vi "_Hightlight CSM Scripts(StringConstant).vi"(11 "reference out":refnum<vi>) -> (0 "error out":errorcluster)   [LabVIEW 2017]
uses:
  Communicable State Machine.lvlib
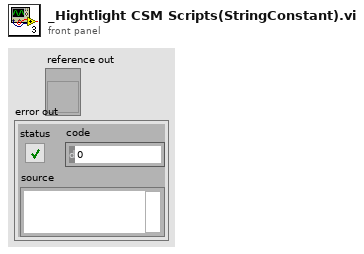
[diagram p1: front panel]
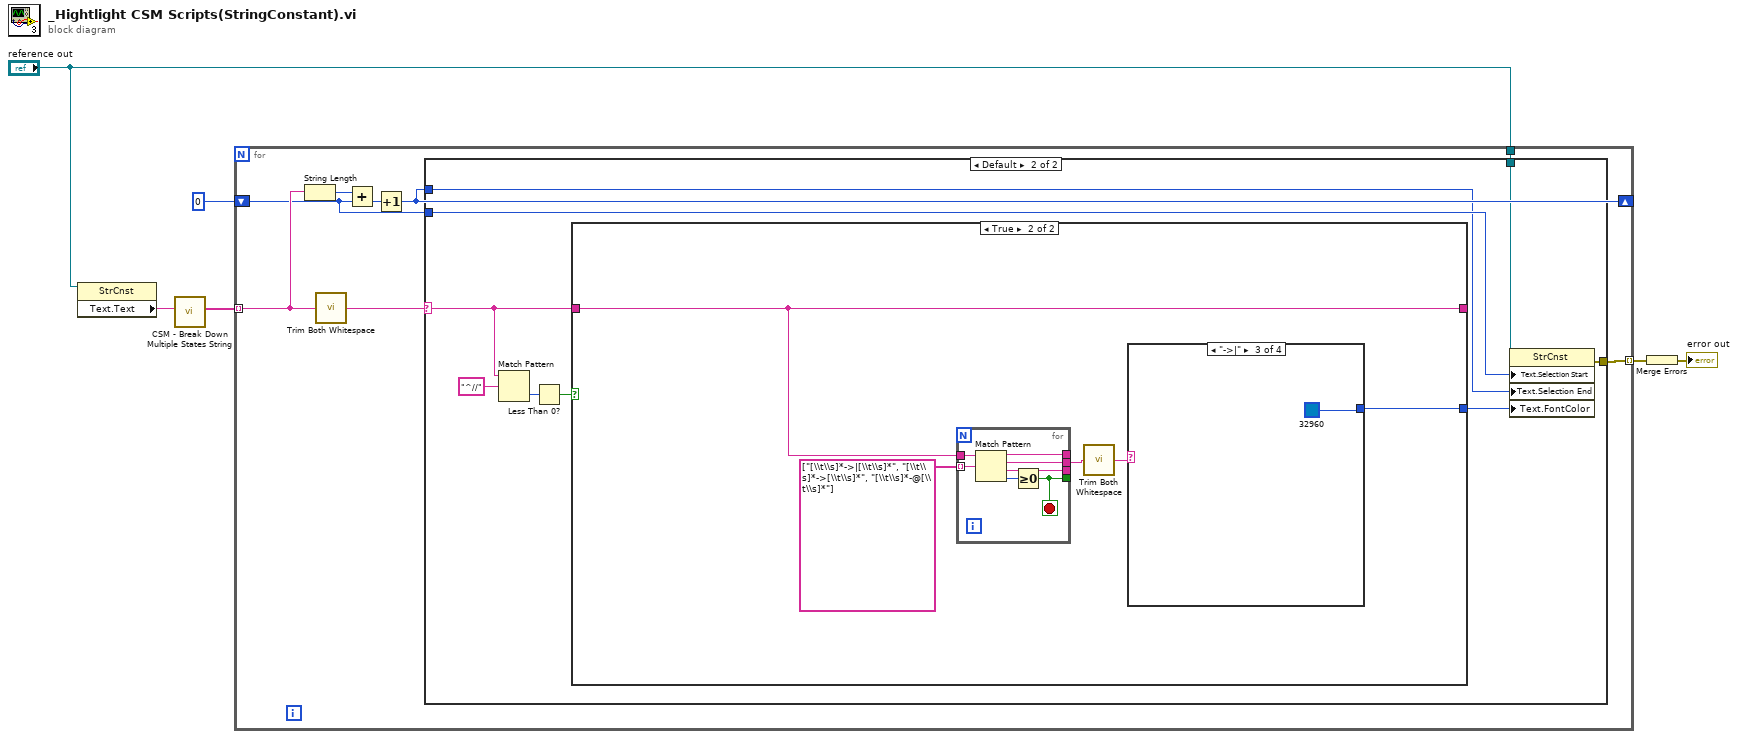
[diagram p0: block diagram]
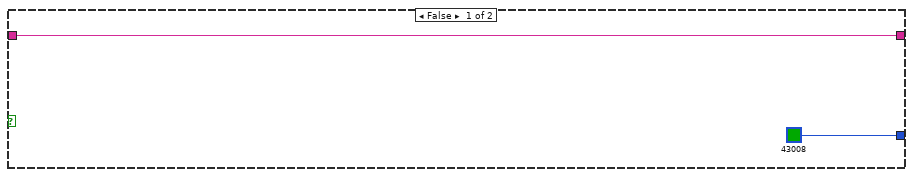
[diagram p3: hidden frame]
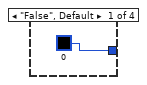
[diagram p4: hidden frame]
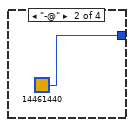
[diagram p5: hidden frame]
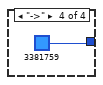
[diagram p6: hidden frame]
diagram:
  n1 = property class="StrCnst"(reference="reference out") -> ("Text.Text"=w4:string)  [unwired: 1 in, 2 out]
  n2 = call "CSM - Break Down Multiple States String.vi"("States"=w4) -> ("Multiple States"=w6:string[])  [unwired: 10 in]
  n3 = for {
    tunnel: w6 -> [w12] mode=indexing
    shift-right: [w8] -> _
    shift-left: u32 0 ("Text.Selection:Start") -> [w10]
    tunnel: "reference out" -> [w11]
    tunnel: [w7] -> w2 mode=indexing
    n4 = String Length(string=w12) -> (length=w13:i32)
    n5 = call "Trim Both Whitespace.vi"("string"=w12) -> ("trimmed string"=w14:string)  [unwired: 1 in]
    n6 = Add(x=w13, y=w10) -> (x+y=w9:u32)
    n7 = Increment(x=w9) -> (x+1=w8:u32)
    n8 = case shown="Default" w14 {
      selector: w14 -> [_ w21]
      tunnel: w11 -> [_ w19]
      tunnel: w10 -> [_ w18]
      tunnel: w8 -> [_ w17]
      tunnel: [_ w15] -> w7
      frame "" {
      }
      frame Default {
        n9 = Match Pattern(string=w21, regular expression="^//") -> (offset past match=w23:i32)  [unwired: 1 in, 3 out]
        n10 = Less Than 0?(x=w23) -> (x < 0?=w20:bool)
        n11 = case shown="True" w20 {
          tunnel: [w25 w28] -> _
          tunnel: w21 -> [w25 w28]
          tunnel: [u32 43008 w27] -> w16
          frame False {
          }
          frame True {
            n12 = for {
              tunnel: w28 -> [w41]
              tunnel: string[] ["[\\t\\s]*->|[\\t\\s]*", "[\\t\\s]*->[\\t\\s]*", "[\\t\\s]*-@[\\t\\s]*"] -> [w40] mode=indexing
              tunnel: [w38] -> _
              tunnel: [w37] -> _
              tunnel: [w36] -> w29
              tunnel: [w35] -> _
              stop <- w38 stop-if-true
              n13 = Match Pattern(string=w41, regular expression=w40) -> (before substring=w37:string, match substring=w36:string, after substring=w35:string, offset past match=w39:i32)  [unwired: 1 in]
              n14 = Greater Or Equal To 0?(x=w39) -> (x >= 0?=w38:bool)
            }
            n15 = call "Trim Both Whitespace.vi"("string"=w29) -> ("trimmed string"=w26:string)  [unwired: 1 in]
            n16 = case shown="\"->|\"" w26 {
              tunnel: [u32 0 u32 14461440 u32 32960 u32 3381759] -> w27
              frame "False", Default {
              }
              frame "-@" {
              }
              frame "->|" {
              }
              frame "->" {
              }
            }
          }
        }
        n17 = property class="StrCnst"(reference=w19, "Text.Selection Start"=w18, "Text.Selection End"=w17, "Text.FontColor"=w16) -> (error out=w15:errorcluster)  [unwired: 1 in, 1 out]
      }
    }
  }
  n18 = Merge Errors(w2) -> (→"error out":errorcluster)
